vi "Validate Parameters.vi"(8 "error in (no error)":errorcluster, 11 "SigMan in":refnum<class "SignalManager.lvclass">) -> (0 "error out":errorcluster, 3 "SigMan out":refnum<class "SignalManager.lvclass">)   [LabVIEW 2015, in "SignalManager.lvclass"]
uses:
  SignalManager.lvclass
  SignalManager.lvclass/SignalManager.ctl
  Channel/Channel.lvclass/Channel.ctl
  Channel/Read Destination.vi
  Channel/Read Name.vi
  Channel/Channel.lvclass
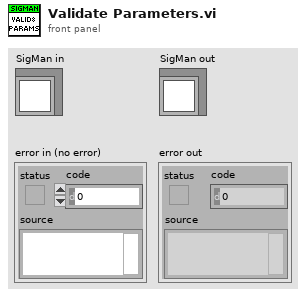
[diagram p1: front panel]
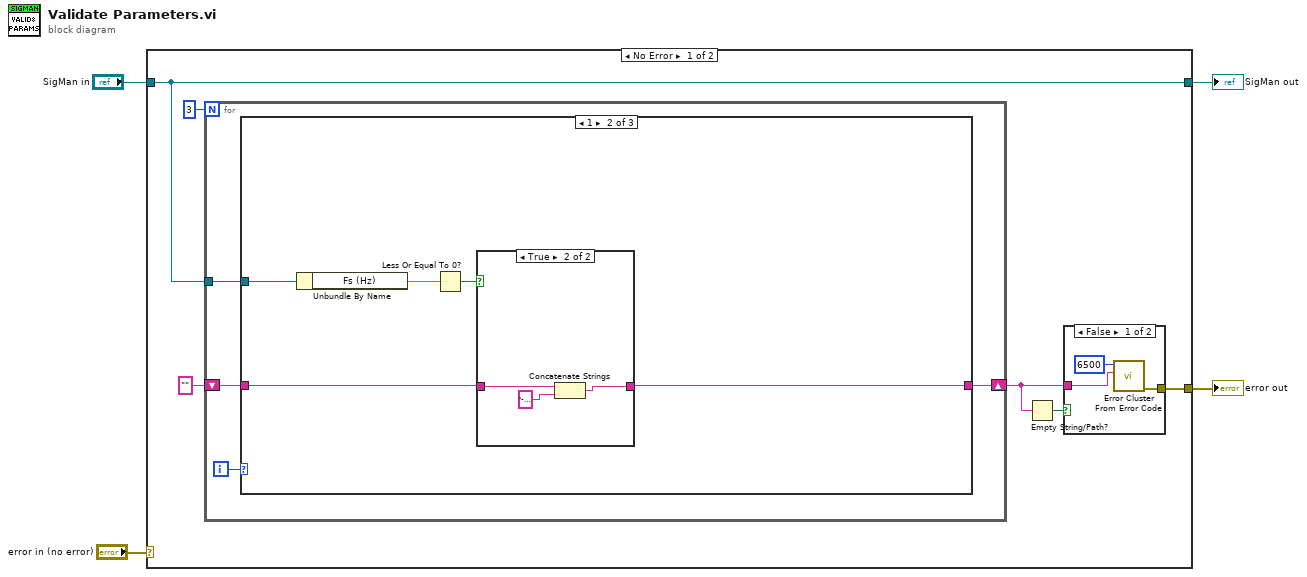
[diagram p0: block diagram]
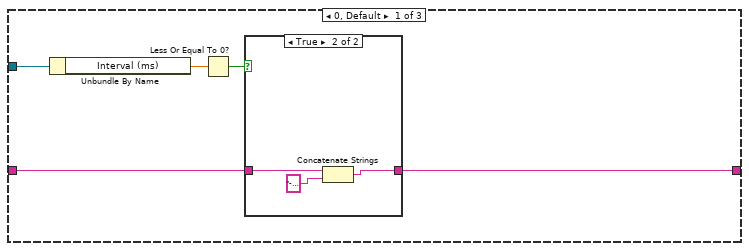
[diagram p3: hidden frame]
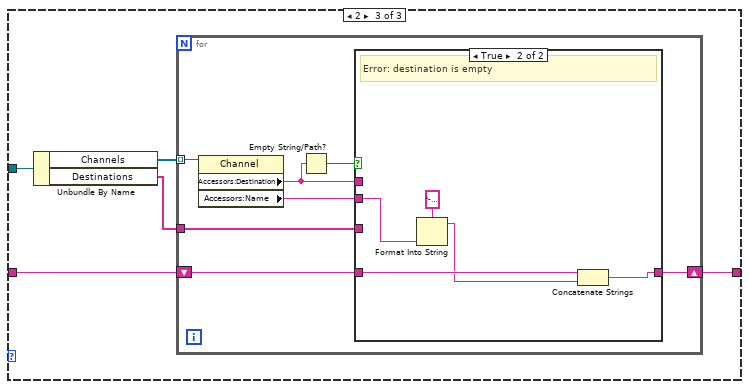
[diagram p6: hidden frame]
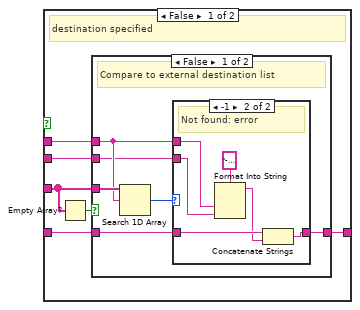
[diagram p7: hidden frame]
diagram:
  n1 = case shown="No Error" "error in (no error)" {
    selector: "error in (no error)" -> [_ w74]
    tunnel: [w5 w74] -> w3
    tunnel: [w8 w73] -> w1
    tunnel: "SigMan in" -> [w8 w73]
    frame No Error {
      n2 = for {
        N: 3 -> [_]
        shift-right: [w15] -> w7
        shift-left: "" -> [w16]
        tunnel: w8 -> [w17]
        i -> [w14]
        n3 = case shown="1" w14 {
          tunnel: w17 -> [w22 w31 w40]
          tunnel: w16 -> [w20 w29 w38]
          tunnel: [w19 w28 w37] -> w15
          frame 0, Default {
            n4 = Unbundle By Name(w22) -> ("Interval (ms)"=w18:dbl)
            n5 = Less Or Equal To 0?(x=w18) -> (x <= 0?=w21:bool)
            n6 = case shown="True" w21 {
              tunnel: w20 -> [w23 w26]
              tunnel: [w23 w25] -> w19
              frame False {
              }
              frame True {
                n7 = Concatenate Strings(w26, "--Interval must be >0\n" ("format string")) -> (w25:string)
              }
            }
          }
          frame 1 {
            n8 = Unbundle By Name(w31) -> ("Fs (Hz)"=w27:dbl)
            n9 = Less Or Equal To 0?(x=w27) -> (x <= 0?=w30:bool)
            n10 = case shown="True" w30 {
              tunnel: w29 -> [w32 w35]
              tunnel: [w32 w34] -> w28
              frame False {
              }
              frame True {
                n11 = Concatenate Strings(w35, "--Sampling rate must be >0\n" ("format string")) -> (w34:string)
              }
            }
          }
          frame 2 {
            n12 = Unbundle By Name(w40) -> ("Channels"=w39:refnum<class "Channel.lvclass">[], "Destinations"=w36:string[])
            n13 = for {
              tunnel: w39 -> [w47] mode=indexing
              shift-right: [w42] -> w37
              shift-left: w38 -> [w43]
              tunnel: w36 -> [w44]
              n14 = property class="Channel"(reference=w47) -> ("Accessors:Destination"=w46:string, "Accessors:Name"=w41:string)  [unwired: 1 in, 2 out]
              n15 = Empty String/Path?(string/path=w46) -> (empty?=w45:bool)
              n16 = case shown="True" w45 {
                tunnel: w46 -> [w50 _]
                tunnel: w44 -> [w51 _]
                tunnel: w43 -> [w53 w72]
                tunnel: [w48 w71] -> w42
                tunnel: w41 -> [w49 w69]
                frame False {
                  # "destination specified"
                  n17 = Empty Array?(array=w51) -> (empty?=w52:bool)
                  n18 = case shown="False" w52 {
                    tunnel: w53 -> [w55 w67]
                    tunnel: w51 -> [w59 _]
                    tunnel: w50 -> [w57 _]
                    tunnel: w49 -> [w56 _]
                    tunnel: [w54 w67] -> w48
                    frame False {
                      # "Compare to external destination list"
                      n19 = Search 1D Array(1D array=w59, element=w57) -> (index of element=w58:i32)  [unwired: 1 in]
                      n20 = case shown="-1" w58 {
                        tunnel: w57 -> [_ w61]
                        tunnel: w56 -> [_ w62]
                        tunnel: w55 -> [w60 w65]
                        tunnel: [w60 w64] -> w54
                        frame 0, Default {
                          # "Found: OK"
                        }
                        frame -1 {
                          # "Not found: error"
                          n21 = Format Into String(format string="--Channel '%s': invalid destination '%s'\n", w61, w62) -> (resulting string=w63:string)  [unwired: 2 in, 1 out]
                          n22 = Concatenate Strings(w65, w63) -> (w64:string)
                        }
                      }
                    }
                    frame True {
                      # "no externally-imposed destination list"
                    }
                  }
                }
                frame True {
                  # "Error: destination is empty"
                  n23 = Format Into String(format string="--Channel '%s': no destination specified\n", w69) -> (resulting string=w68:string)  [unwired: 2 in, 1 out]
                  n24 = Concatenate Strings(w72, w68) -> (w71:string)
                }
              }
            }
          }
        }
      }
      n25 = Empty String/Path?(string/path=w7) -> (empty?=w6:bool)
      n26 = case shown="False" w6 {
        tunnel: w7 -> [w12 _]
        tunnel: [w11 _] -> w5
        frame False {
          n27 = call <vilib>:"Error Cluster From Error Code.vi"("error message (\"\")"=w12, "error code (0)"=6500) -> ("error out"=w11:errorcluster)  [unwired: 7 in]
        }
        frame True {
        }
      }
    }
    frame Error {
    }
  }
  "error out" <- w3
  "SigMan out" <- w1
